vi "Data_Set Path.vi"(8 "error in (no error)":errorcluster, 9 "Path":path, 10 "Time Stamp":timestamp, 11 "variant":variant) -> (0 "error out":errorcluster, 3 "variant out":variant)   [LabVIEW 2015, in "Exposure Process.lvlib"]
uses:
  Exposure Process.lvlib
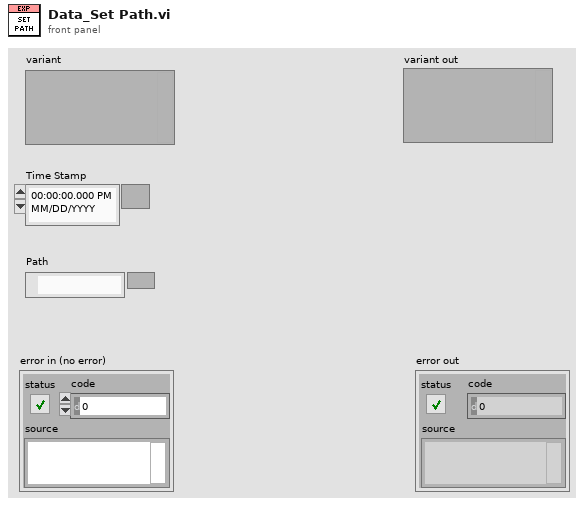
[diagram p1: front panel]
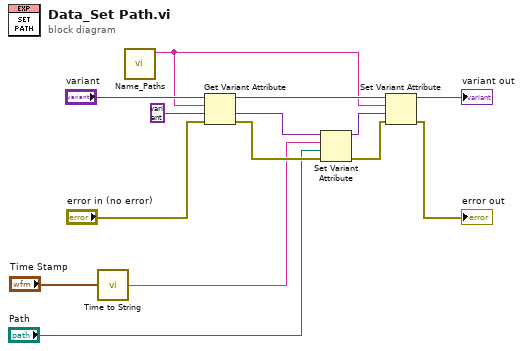
[diagram p0: block diagram]
diagram:
  n1 = call "Time to String.vi"("Time Stamp"="Time Stamp") -> ("date/time string"=w1:string)
  n2 = call "Name_Paths.vi"() -> ("Name"=w6:string)  [unwired: 11 in]
  n3 = Get Variant Attribute(Variant="variant", name=w6, default value (empty Variant)=variant, error in="error in (no error)") -> (duplicate Variant=w8:variant, value=w11:variant, error out=w10:errorcluster)  [unwired: 1 out]
  n4 = Set Variant Attribute(Variant=w11, name=w1, value="Path", error in=w10) -> (Variant out=w7:variant, error out=w5:errorcluster)  [unwired: 1 out]
  n5 = Set Variant Attribute(Variant=w8, name=w6, value=w7, error in=w5) -> (Variant out=→"variant out":variant, error out=→"error out":errorcluster)  [unwired: 1 out]
